vi "Write FileName.vi"(8 "error in (no error)":errorcluster, 10 "FileName":string, 11 "Project in":refnum<class "Project.lvclass">) -> (0 "error out":errorcluster, 3 "Project out":refnum<class "Project.lvclass">)   [LabVIEW 2015, in "Project.lvclass"]
uses:
  Project.lvclass
  Project.lvclass/Project.ctl
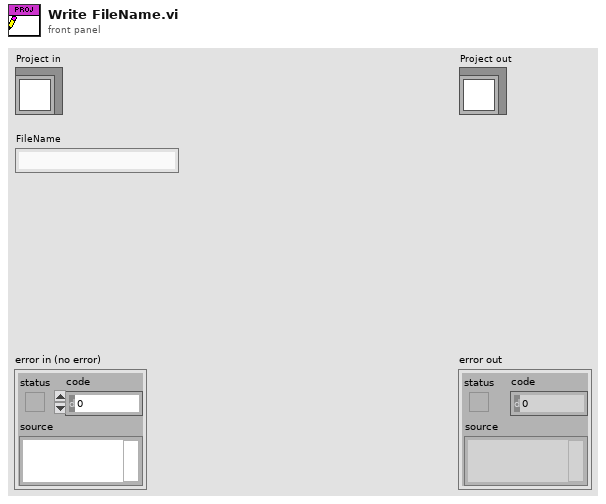
[diagram p1: front panel]
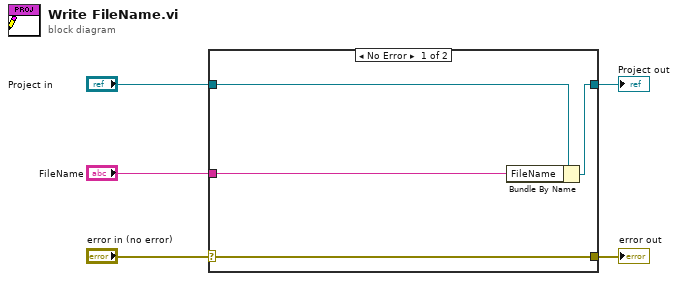
[diagram p0: block diagram]
diagram:
  n1 = case shown="No Error" "error in (no error)" {
    selector: "error in (no error)" -> [w9 w10]
    tunnel: [w9 w10] -> w4
    tunnel: [w7 w11] -> w2
    tunnel: "Project in" -> [w8 w11]
    tunnel: "FileName" -> [w6 _]
    frame No Error {
      n2 = Bundle By Name(cluster=w8, "FileName"=w6) -> (w7:refnum<class "Project.lvclass">)
    }
    frame Error {
    }
  }
  "error out" <- w4
  "Project out" <- w2
